vi "Create Event.vi"(8 "error in (no error)":errorcluster, 11 "Messaging in":refnum<class "Messaging.lvclass">) -> (0 "error out":errorcluster, 3 "Messaging out":refnum<class "Messaging.lvclass">)   [LabVIEW 2023, in "Messaging.lvclass"]
uses:
  Messaging.lvclass
  Messaging.lvclass/Messaging.ctl
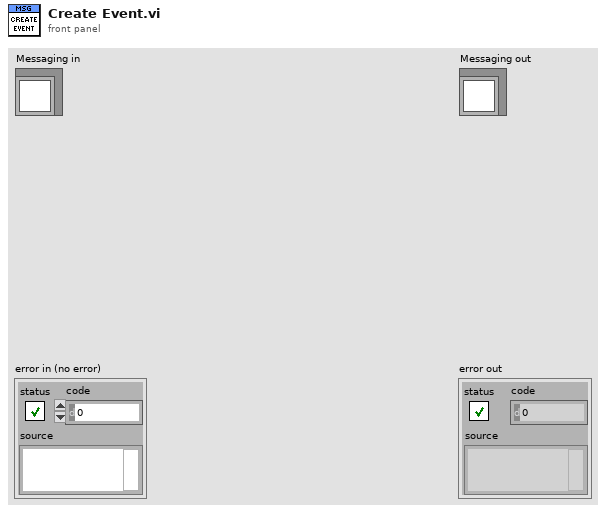
[diagram p1: front panel]
types:
  T1 = typedef "Msg.Event.Ref.ctl" = refnum<user-event>
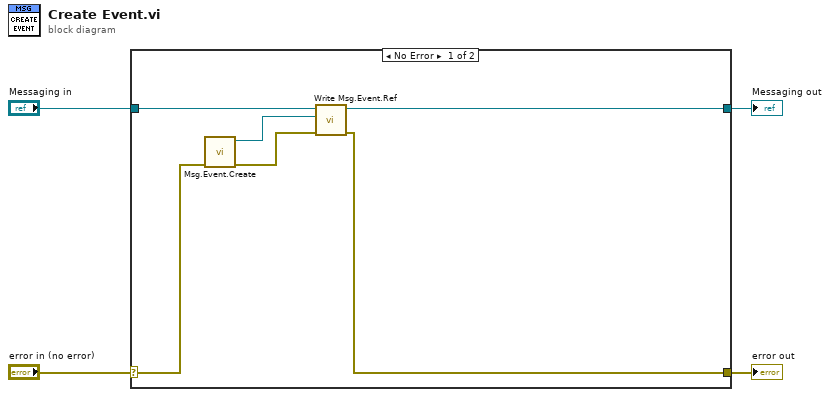
[diagram p0: block diagram]
diagram:
  n1 = case shown="No Error" "error in (no error)" {
    selector: "error in (no error)" -> [w8 w12]
    tunnel: [w6 w12] -> w3
    tunnel: [w5 w11] -> w1
    tunnel: "Messaging in" -> [w10 w11]
    frame No Error {
      n2 = call "Msg.Event.Create.vi"("Error (in)"=w8) -> ("Error (out)"=w7:errorcluster, "Msg.Event.Data (out)"=w9:T1)  [unwired: 9 in]
      n3 = call-dynamic "Write Msg.Event.Ref.vi"("error in (no error)"=w7, "Msg.Event.Ref"=w9, "Messaging in"=w10) -> ("error out"=w6:errorcluster, "Messaging out"=w5:refnum<class "Messaging.lvclass">)  [unwired: 7 in]
    }
    frame Error {
    }
  }
  "error out" <- w3
  "Messaging out" <- w1
